vi "nodeFromPubSub.vi"(2 "PubSub in":T1) -> (0 "Node":cluster{"Name":string, "URI":string})   [LabVIEW 2013, in "ROS_Master.lvclass"]
uses:
  <userlib>/ROS_Master/ROS_Master.lvclass
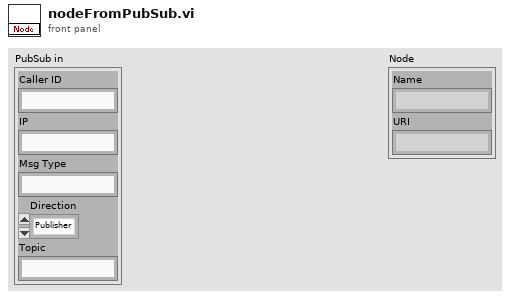
[diagram p1: front panel]
types:
  T1 = cluster{"Caller ID":string, "IP":string, "Msg Type":string, "Direction":enum16{"Publisher", "Subscriber"}, "Topic":string}
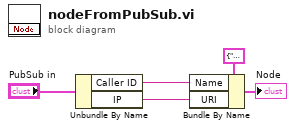
[diagram p0: block diagram]
diagram:
  n1 = Unbundle By Name("PubSub in") -> ("Caller ID"=w3:string, "IP"=w2:string)
  n2 = Bundle By Name(cluster=cluster{"Name":string, "URI":string} {"Name"="", "URI"=""} ("Node"), "Name"=w3, "URI"=w2) -> (→"Node":cluster{"Name":string, "URI":string})
